vi "Write cell.vi"(8 "error in (no error)":errorcluster, 10 "cell":u8, 11 "Filter Step in":refnum<class "Filter Step.lvclass">) -> (0 "error out":errorcluster, 3 "Filter Step out":refnum<class "Filter Step.lvclass">)   [LabVIEW 2016, in "Controller.lvlib" / "Filter Step.lvclass"]
uses:
  Filter Step.lvclass
  Filter Step.lvclass/Filter Step.ctl
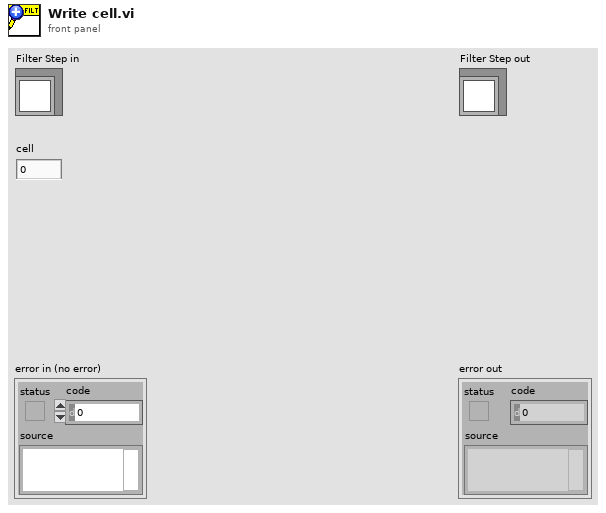
[diagram p1: front panel]
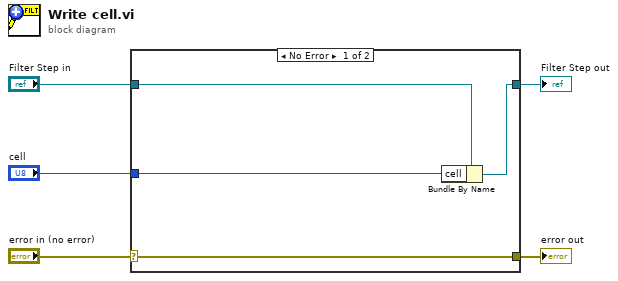
[diagram p0: block diagram]
diagram:
  n1 = case shown="No Error" "error in (no error)" {
    selector: "error in (no error)" -> [w9 w10]
    tunnel: [w9 w10] -> w4
    tunnel: [w7 w11] -> w2
    tunnel: "Filter Step in" -> [w8 w11]
    tunnel: "cell" -> [w6 _]
    frame No Error {
      n2 = Bundle By Name(cluster=w8, "cell"=w6) -> (w7:refnum<class "Filter Step.lvclass">)
    }
    frame Error {
    }
  }
  "error out" <- w4
  "Filter Step out" <- w2
